vi "ExCircNframeBigBufBin2xCas.vi"() -> ()   [LabVIEW 2010]
panel:
  in  "ADC Gain":u32
  out "ADC Speed (Khz)":u32
  in  "Fast ADC":bool
  in  "Avalanche Gain\nOnly valid for \nport 0":dbl format="%.2f"
  in  "ReadOut Port":u32 max=1 step=1
  in  "OverLap Mode":bool
  out "ready to \nstart":bool
  in  "Start collection":bool
  in  "Timing Mode":u32(ring)=1 items=["N/A", "Timed Mode/Free run", "Trigger First (only PM)", "Strobed/Ext Sync", "Bulb Mode (PM only)", "Variable Timed mode (PM only)", "Flash Mode (only some PM)"]
  in  "Number of Images":u32=1 min=1 step=1
  in  "Temperature":dbl=-10.0 format="%.2f"
  in  "Exposure":dbl min=0.0 step=0.001 format="%.3f"
  out "error out":errorcluster
  in  "error in (no error)":errorcluster
  # "ExCircNframeBigBufBin2x:\nThis example collects, displays, and saves in \na .spe file the number of images selected. This \nexample requires the camera have circular \nbuffers capability. \nFirst this example creates an array of image \nhandles. It then collects data into this array.\nFinally it displays and saves all the images."
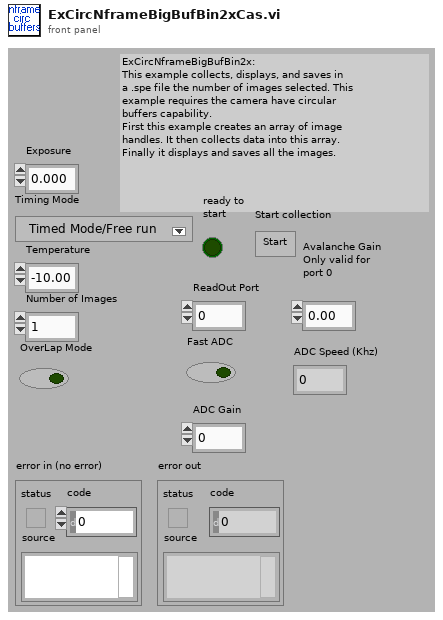
[diagram p1: front panel]
types:
  T1 = cluster{"acquire focus mode":u32, "Exposure":dbl, "Number of Images":u32, "Software accumulation":u32}
  T2 = cluster{"Camera Handle":u32, "Pulser Handle":u32, "File Handle":u32, "Display Handle":u32, "Image Handle":u32}
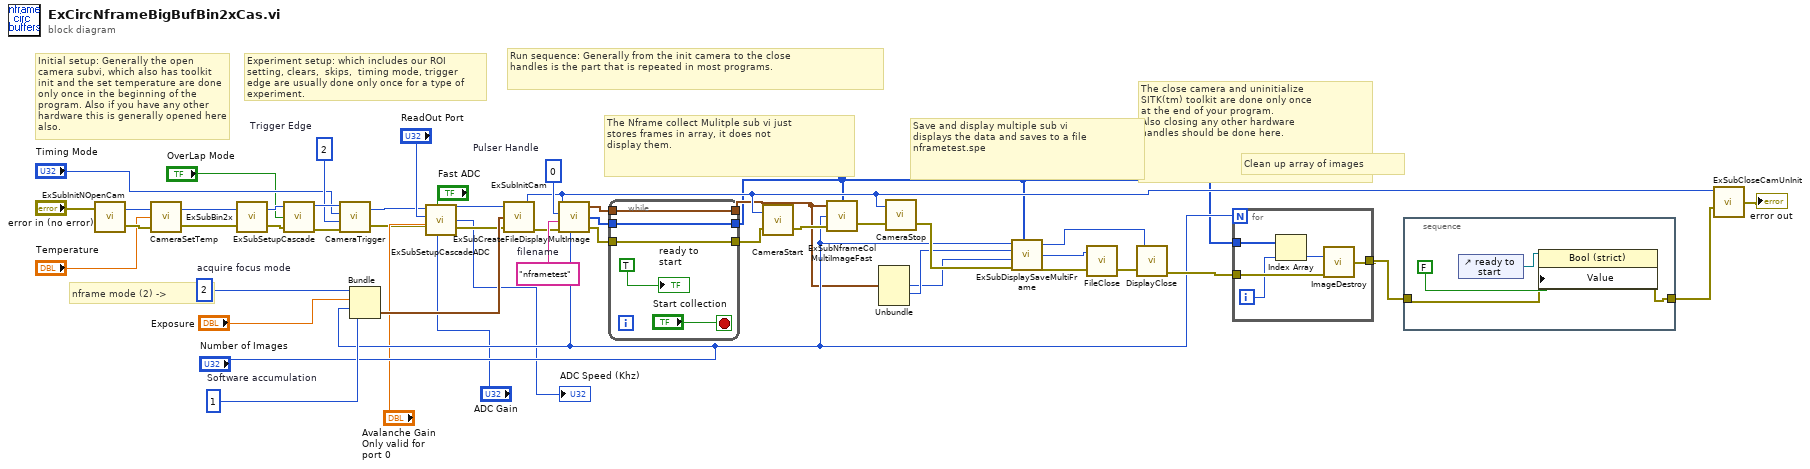
[diagram p0: block diagram]
diagram:
  w40 = u32 0  # Pulser Handle
  w41 = u32 2  # Trigger Edge
  w43 = u32 2  # acquire focus mode
  w42 = u32 1  # Software accumulation
  w50 = "nframetest"  # filename
  # "Clean up array of images"
  # "Save and display multiple sub vi\ndisplays the data and saves to a file\nnframetest.spe"
  # "The Nframe collect Mulitple sub vi just \nstores frames in array, it does not \ndisplay them."
  # "The close camera and uninitialize\nSITK(tm) toolkit are done only once\nat the end of your program.\nAlso closing any other hardware \nhandles should be done here."
  # "Run sequence: Generally from the init camera to the close \nhandles is the part that is repeated in most programs."
  # "Experiment setup: which includes our ROI setting, clears,  skips,  timing mode, trigger edge are usually done only once for a type of experiment."
  # "Initial setup: Generally the open camera subvi, which also has toolkit init and the set temperature are done only once in the beginning of the program. Also if you have any other hardware this is generally opened here also."
  # "nframe mode (2) ->"
  n1 = call "ExSubInitNOpenCam.vi"("error in (no error)"="error in (no error)") -> ("Camera Handle"=w36:u32, "error out"=w35:errorcluster)
  n2 = call <userlib>:"CameraSetTemp.vi"("error in (no error)"=w35, "Temperature"="Temperature", "Camera Handle"=w36) -> ("error out"=w38:errorcluster, "Camera Handle"=w37:u32)
  n3 = call "ExSubBin2x.vi"("error in (no error)"=w38, "Camera Handle"=w37) -> ("error out"=w32:errorcluster, "Camera Handle"=w33:u32)
  n4 = call "ExSubSetupCascade.vi"("error in (no error)"=w32, "OverLap Mode"="OverLap Mode", "Camera Handle"=w33) -> ("error out"=w44:errorcluster, "Camera Handle"=w45:u32)
  n5 = call <userlib>:"CameraTrigger.vi"("error in"=w44, "Trigger Edge"=w41, "Timing Mode"="Timing Mode", "Camera Handle"=w45) -> ("error out"=w2:errorcluster, "Camera Handle"=w1:u32)
  n6 = Bundle("acquire focus mode"=w43, "Exposure"="Exposure", "Number of Images"="Number of Images", "Software accumulation"=w42) -> (w47:T1)  [unwired: 1 in]
  n7 = call "ExSubSetupCascadeADC.vi"("Camera Handle"=w1, "Fast ADC"="Fast ADC", "ReadOut Port"="ReadOut Port", "Avalanche Gain\nOnly valid for \nport 0"="Avalanche Gain\nOnly valid for \nport 0", "ADC Gain"="ADC Gain", "error in (no error)"=w2) -> ("Camera Handle"=w8:u32, "ADC Speed (Khz)"=→"ADC Speed (Khz)":u32, "error out"=w9:errorcluster)
  n8 = call "ExSubInitCam.vi"("error in (no error)"=w9, "Camera Information"=w47, "Camera Handle"=w8) -> ("error out"=w46:errorcluster, "Camera Handle"=w30:u32)
  n9 = call "ExSubCreateFileDisplayMultImage.vi"("Camera Handle"=w30, "Pulser Handle"=w40, "File and Display Name"=w50, "error in (no error)"=w46, "Number of Images"="Number of Images") -> ("Handles Out"=w18:T2, "Array"=w14:u32[], "error out"=w16:errorcluster)
  n10 = while {
    tunnel: w18 -> [w55]
    tunnel: [w55] -> w17
    tunnel: w16 -> [w54]
    tunnel: [w54] -> w15
    tunnel: w14 -> [w53]
    tunnel: [w53] -> w13
    stop <- "Start collection" stop-if-true
    "ready to \nstart" <- TRUE
  }
  n11 = call <userlib>:"CameraStart.vi"("error in"=w15, "Camera Handle"=w30) -> ("error out"=w39:errorcluster)  [unwired: 1 out]
  n12 = call "ExSubNframeColMultiImageFast.vi"("image handles"=w13, "error in (no error)"=w39, "Number of Images"="Number of Images", "Handle Cluster"=w17) -> ("error out"=w31:errorcluster)  [unwired: 1 out]
  n13 = Unbundle(w17) -> ("File Handle"=w25:u32, "Display Handle"=w26:u32)  [unwired: 3 out]
  n14 = call <userlib>:"CameraStop.vi"("error in"=w31, "Camera Handle"=w30) -> ("error out"=w27:errorcluster)  [unwired: 1 out]
  n15 = call "ExSubDisplaySaveMultiFrame.vi"("Number of Images"="Number of Images", "Display Handle"=w26, "file handle"=w25, "error in (no error)"=w27, "Data handles"=w13) -> ("Display Handle"=w20:u32, "file Handle"=w21:u32, "error out"=w22:errorcluster)
  n16 = call <userlib>:"FileClose.vi"("error in"=w22, "File Handle"=w21) -> ("error out"=w24:errorcluster)
  n17 = call <userlib>:"DisplayClose.vi"("error in"=w24, "Display Handle"=w20) -> ("error out"=w23:errorcluster)
  n18 = for {
    N: "Number of Images" -> [_]
    tunnel: w23 -> [w60]
    tunnel: [w59] -> w12
    tunnel: w13 -> [w57]
    i -> [w58]
    n19 = Index Array(array=w57, index=w58) -> (element=w56:u32)
    n20 = call <userlib>:"ImageDestroy.vi"("error in"=w60, "Data handle"=w56) -> ("error out"=w59:errorcluster)
  }
  n21 = stacked-sequence {
    tunnel: w12 -> [w62]
    tunnel: [w61] -> w11
    frame #0 {
      n22 = control-ref of="ready to \nstart"() -> (w64:refnum<vi>)
      n23 = property class="Bool (strict)"(reference=w64, error in=w62, "Value"=FALSE) -> (error out=w61:errorcluster)  [unwired: 1 out]
    }
  }
  n24 = call "ExSubCloseCamUnInit.vi"("error in (no error)"=w11, "Camera Handle"=w30) -> ("error out"=→"error out":errorcluster)
